vi "Music File Manager(Main).vi"(9 "Samples Per Channel":i32=10) -> ()   [LabVIEW 2014]
uses:
  Controls/File Operation.ctl
  Controls/Track (File) References.ctl
  Controls/4 Track Audio.ctl
  Controls/Audio In.ctl
  Controls/Track Enable.ctl
panel:
  out "4-Track Audio 2":T1
  in  "Track Enable Read":T3
  in  "Number Of Elements to Read":i64
  in  "Read Position":i64
  in  "Write Position":i64
  in  "Track Enable":T3={"Track_1 _Enable "=TRUE, "Track_2 _Enable "=FALSE, "Track_3 _Enable "=TRUE, "Track_4 _Enable "=FALSE}
  in  "4-Track Audio":T1
  in  "Stop Main":bool
  in  "Track (File) Refereces In":T4
  out "Track (File) Refereces Out":T4
  out "Error Out":errorcluster
  in  "Error In":errorcluster
  in  "File Operation":T5
  in  "Track Name":string
  # "WRITING TEST"
  # "READING TEST"
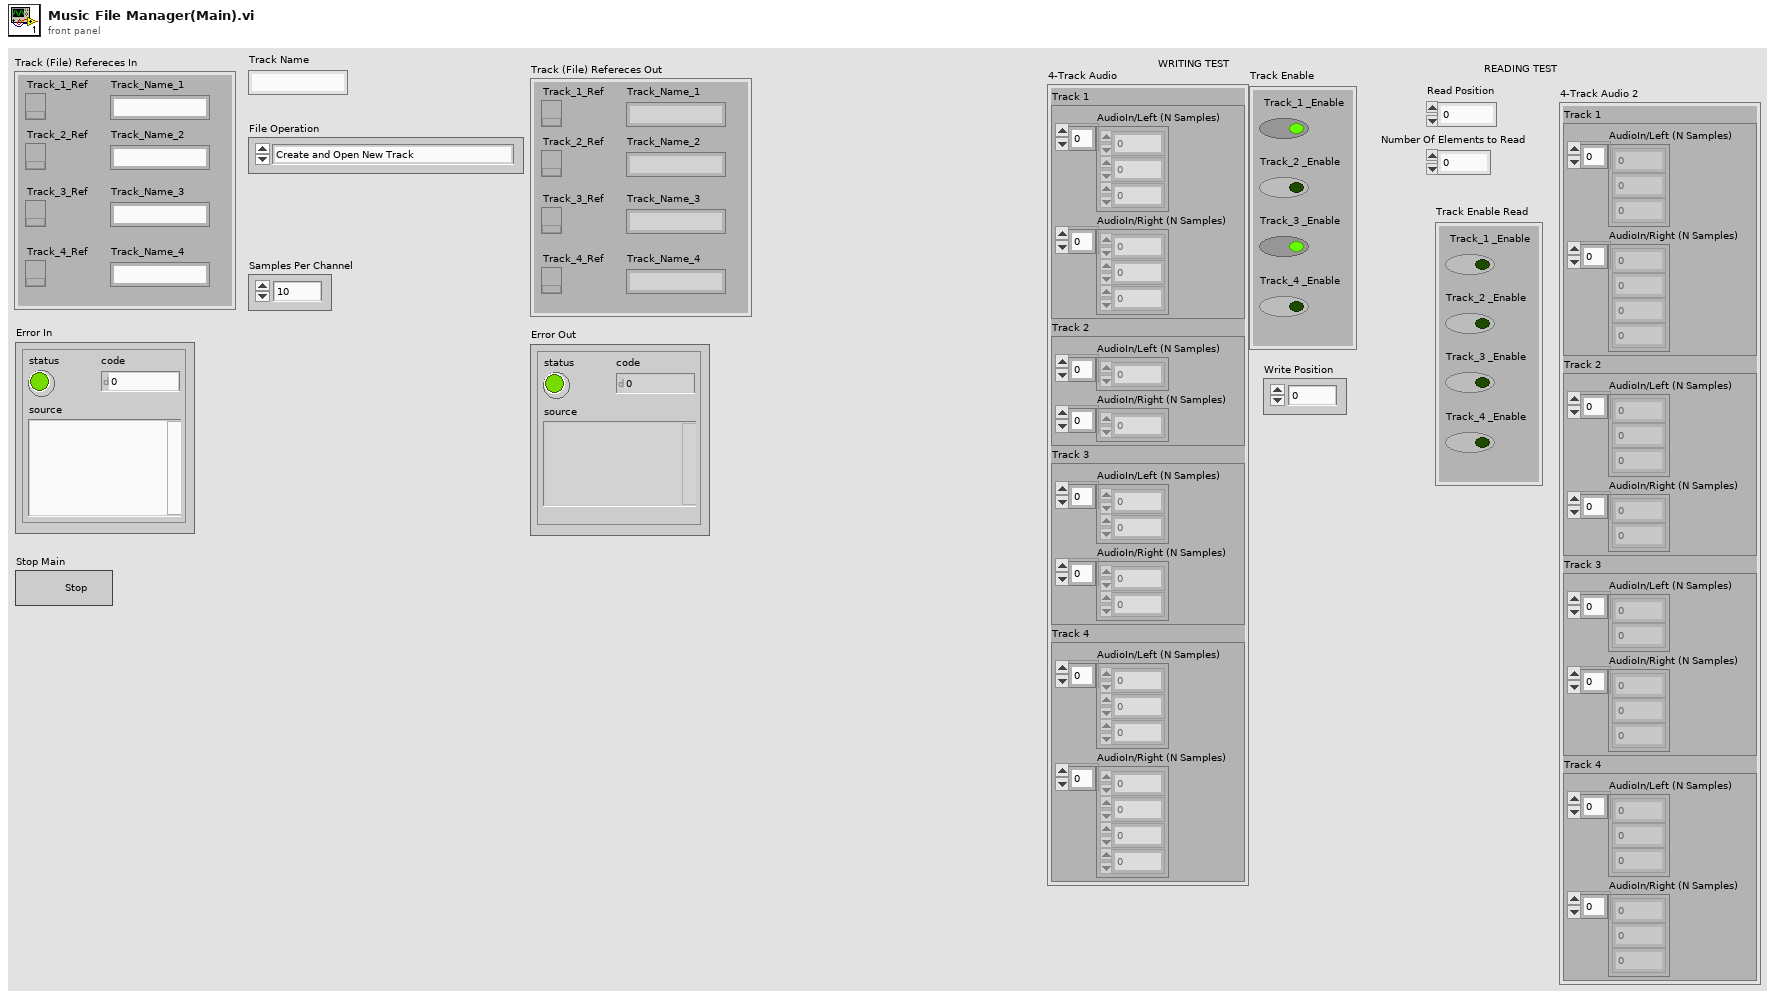
[diagram p1: front panel]
types:
  T1 = typedef "4 Track Audio.ctl" = cluster{"Track 1":T2, "Track 2":T2, "Track 3":T2, "Track 4":T2}
  T2 = typedef "Audio In.ctl" = cluster{"AudioIn/Left (N Samples)":i16[], "AudioIn/Right (N Samples)":i16[]}
  T3 = typedef "Track Enable.ctl" = cluster{"Track_1 _Enable ":bool, "Track_2 _Enable ":bool, "Track_3 _Enable ":bool, "Track_4 _Enable ":bool}
  T4 = typedef "Track (File) References.ctl" = cluster{"Track_1_Ref":refnum<k34>, "Track_2_Ref":refnum<k34>, "Track_3_Ref":refnum<k34>, "Track_4_Ref":refnum<k34>, "Track_Name_1":string, "Track_Name_2":string, "Track_Name_3":string, "Track_Name_4":string}
  T5 = typedef "File Operation.ctl" = enum16{"Create and Open New Track", "Open Existing Track", "Read Track", "Write Track", "Save Track", "Close Track"}
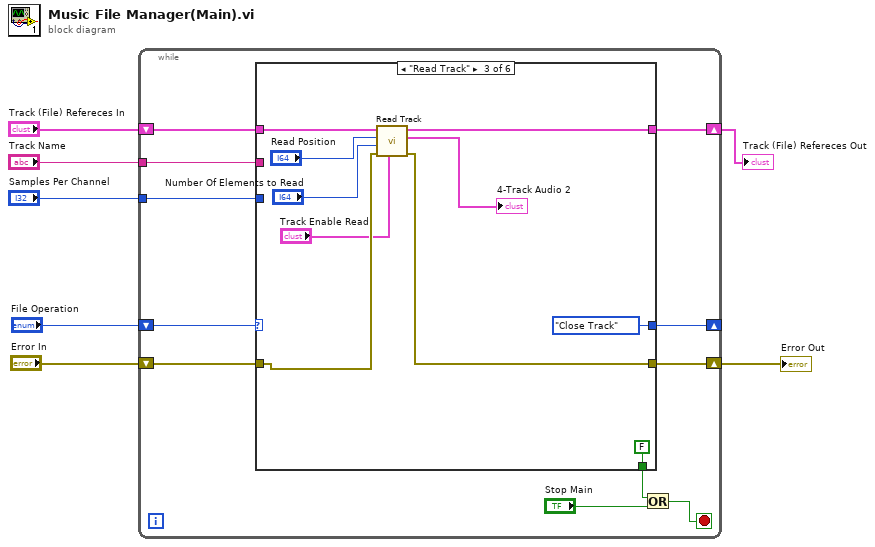
[diagram p0: block diagram]
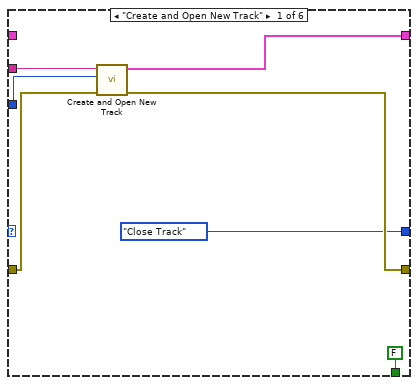
[diagram p2: hidden frame]
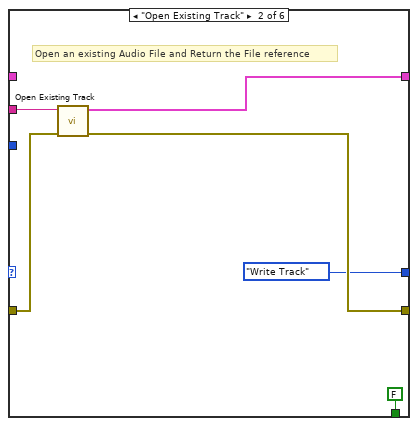
[diagram p3: hidden frame]
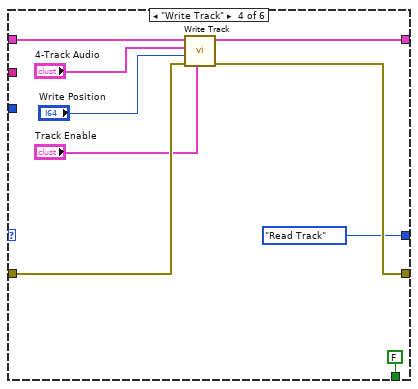
[diagram p4: hidden frame]
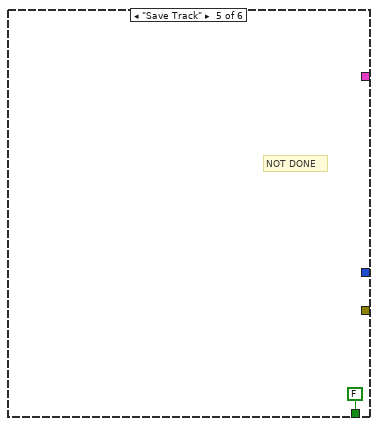
[diagram p5: hidden frame]
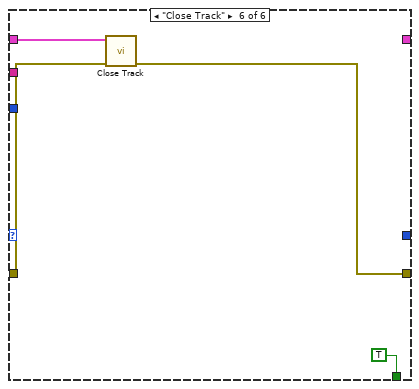
[diagram p6: hidden frame]
diagram:
  n1 = while {
    tunnel: "Track Name" -> [w16]
    tunnel: "Samples Per Channel" -> [w15]
    shift-right: [w14] -> w3
    shift-left: "Track (File) Refereces In" -> [w13]
    shift-right: [w12] -> w1
    shift-left: "Error In" -> [w17]
    shift-right: [w11] -> _
    shift-left: "File Operation" -> [w18]
    stop <- w10 stop-if-true
    n2 = case shown="\"Read Track\"" w18 {
      tunnel: w17 -> [w24 w30 w37 w49 _ w54]
      tunnel: w16 -> [w25 w31 _ _ _ _]
      tunnel: [w21 w28 w36 w48 _ w53] -> w12
      tunnel: w15 -> [w23 _ _ _ _ _]
      tunnel: [w22 w29 w34 w45 _ _] -> w14
      tunnel: w13 -> [_ _ w40 w46 _ w55]
      tunnel: [File_Operation."Close Track" ("File Operation") File_Operation."Write Track" ("File Operation") File_Operation."Close Track" ("File Operation") File_Operation."Read Track" ("File Operation") _ _] -> w11
      tunnel: [FALSE ("x") FALSE ("x") FALSE ("x") FALSE ("x") FALSE ("x") TRUE ("x")] -> w8
      frame "Create and Open New Track" {
        n3 = call "Create and Open New Track.vi"("Error In"=w24, "Samples Per Channel"=w23, "Track Name"=w25) -> ("Error Out"=w21:errorcluster, "Track (File) References"=w22:T4)  [unwired: 7 in]
      }
      frame "Open Existing Track" {
        # "Open an existing Audio File and Return the File reference"
        n4 = call "Open Existing Track.vi"("error in (no error)"=w30, "Track Name"=w31) -> ("error out"=w28:errorcluster, "Track (File) References"=w29:T4)  [unwired: 8 in]
      }
      frame "Read Track" {
        n5 = call "Read Track.vi"("Track Enable"="Track Enable Read", "Error In"=w37, "Number Of Elements to Read"="Number Of Elements to Read", "Read Position"="Read Position", "Track (File) References In"=w40) -> ("Error Out"=w36:errorcluster, "4-Track Audio"=→"4-Track Audio 2":T1, "Track (File) References Out"=w34:T4)  [unwired: 4 in]
      }
      frame "Write Track" {
        n6 = call "Write Track.vi"("Track Enable"="Track Enable", "Error In"=w49, "Write Position"="Write Position", "4-Track Audio"="4-Track Audio", "Track (File) References In"=w46) -> ("Error Out"=w48:errorcluster, "Track (File) References Out"=w45:T4)  [unwired: 5 in]
      }
      frame "Save Track" {
        # "NOT DONE"
      }
      frame "Close Track" {
        n7 = call "Close Track.vi"("Error In"=w54, "Track (File) References"=w55) -> ("Error Out"=w53:errorcluster)  [unwired: 9 in]
      }
    }
    n8 = Or(x=w8, y="Stop Main") -> (x .or. y?=w10:bool)
  }
  "Track (File) Refereces Out" <- w3
  "Error Out" <- w1
